vi "okno.vi"(11 "name or relative path":string="Visualisation.vi") -> ()   [LabVIEW 2018]
panel:
  out "Numeric":dbl
  out "Execution:State":T1(ring)
  out "appended path":path
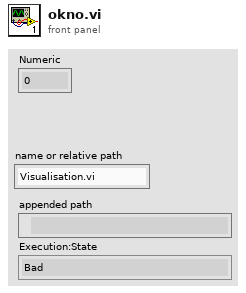
[diagram p1: front panel]
types:
  T1 = enum32{"Bad", "Idle", "Run top level", "Running"}
  T2 = enum32{"Invalid", "Standard", "Closed", "Hidden", "Minimized", "Maximized"}
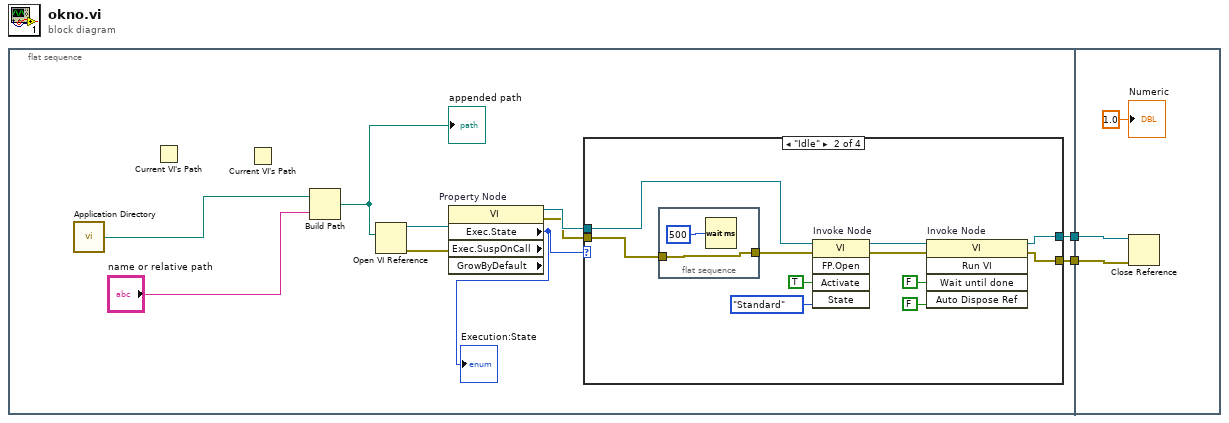
[diagram p0: block diagram]
diagram:
  n1 = flat-sequence {
    tunnel: [w12] -> w2
    tunnel: [w11] -> w1
    tunnel: w2 -> [w33]
    tunnel: w1 -> [w34]
    frame #0 {
      n2 = call <vilib>:"Application Directory.vi"() -> ("Application Directory"=w10:path)
      n3 = Current VI's Path() -> ()  [unwired: 1 out]
      n4 = Current VI's Path() -> ()  [unwired: 1 out]
      n5 = Build Path(base path=w10, name or relative path="name or relative path") -> (appended path=w9:path)
      "appended path" <- w9
      n6 = Open VI Reference(vi path=w9) -> (vi reference=w8:refnum<vi>, error out=w5:errorcluster)  [unwired: 5 in]
      n7 = property on="Property Node" class="VI" props=["Exec.State", "Exec.SuspOnCall", "GrowByDefault"](reference=w8, error in=w5) -> (reference out=w7:refnum<vi>, error out=w6:errorcluster, "Exec.State"=w4:T1)  [unwired: 2 out]
      "Execution:State" <- w4
      n8 = case shown="\"Idle\"" w4 {
        tunnel: [w14 w19 w29 w31] -> w12
        tunnel: [w13 w18 w28 w30] -> w11
        tunnel: w7 -> [w14 w17 w29 w31]
        tunnel: w6 -> [w13 w15 w28 w30]
        frame "Bad", Default {
        }
        frame "Idle" {
          n9 = flat-sequence {
            tunnel: [w27] -> w16
            tunnel: w15 -> [w27]
            frame #0 {
              n10 = Wait (ms)(milliseconds to wait=u32 500) -> ()  [unwired: 1 out]
            }
          }
          n11 = invoke on="Invoke Node" class="VI" method="FP.Open"(reference=w17, error in=w16, "Activate"=TRUE ("Activate?"), "State"=T2."Standard") -> (reference out=w23:refnum<vi>, error out=w22:errorcluster)  [unwired: 1 in, 3 out]
          n12 = invoke on="Invoke Node" class="VI" method="Run VI"(reference=w23, error in=w22, "Wait until done"=FALSE ("Wait Until Done"), "Auto Dispose Ref"=FALSE ("Auto Dispose Reference")) -> (reference out=w19:refnum<vi>, error out=w18:errorcluster)  [unwired: 1 in, 3 out]
        }
        frame "Run top level" {
        }
        frame "Running" {
        }
      }
    }
    frame #1 {
      n13 = Close Reference(reference=w33, error in (no error)=w34) -> ()  [unwired: 1 out]
      "Numeric" <- 1.0 ("Numeric")
    }
  }
